vi "FigureExample.vi"() -> ()   [LabVIEW 2021]
doc: "Example of figures classes."
uses:
  Circle/Circle.lvclass
  Rectangle/Rectangle.lvclass
  Square/Square.lvclass
  Figure/Figure.lvclass
panel:
  out "Canva":picture
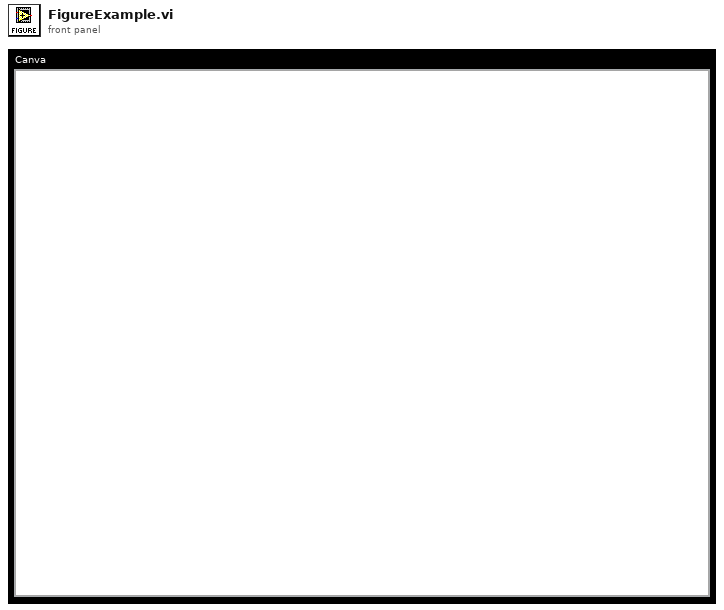
[diagram p1: front panel]
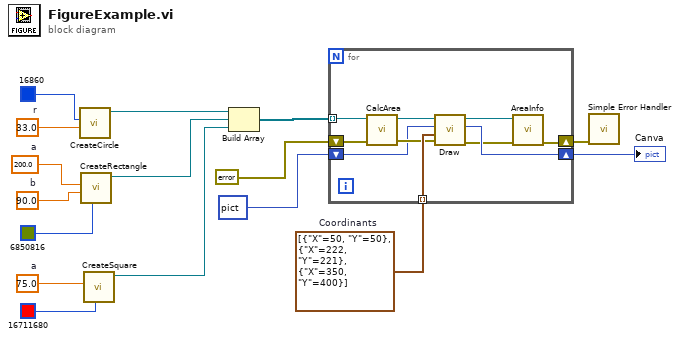
[diagram p0: block diagram]
diagram:
  w3 = cluster{"X":i16, "Y":i16}[] [{"X"=50, "Y"=50}, {"X"=222, "Y"=221}, {"X"=350, "Y"=400}]  # Coordinants
  w10 = 200.0  # a
  w11 = 90.0  # b
  w15 = 33.0  # r
  w16 = 75.0  # a
  n1 = call "CreateCircle.vi"("r"=w15, "Color"=u32 16860) -> ("Circle out"=w9:refnum<class "Circle.lvclass">)  [unwired: 8 in, 1 out]
  n2 = call "CreateRectangle.vi"("Color"=u32 6850816, "b"=w11, "a"=w10) -> ("Rectangle Out"=w8:refnum<class "Rectangle.lvclass">)  [unwired: 7 in, 1 out]
  n3 = call "CreateSquare.vi"("Color"=u32 16711680, "a"=w16) -> ("Square out"=w7:refnum<class "Square.lvclass">)  [unwired: 8 in, 1 out]
  n4 = Build Array(w9, w8, w7) -> (w6:refnum<class "Figure.lvclass">[])
  n5 = for {
    tunnel: w6 -> [w22] mode=indexing
    shift-right: [w26] -> w4
    shift-left: picture data[5B] ("2D Picture In") -> [w19]
    tunnel: w3 -> [w25] mode=indexing
    shift-right: [w18] -> w1
    shift-left: errorcluster {"status"=FALSE, "code"=0, "source"=""} ("Error Out") -> [w17]
    n6 = call-dynamic "CalcArea.vi"("Error In"=w17, "Figure in"=w22) -> ("Error Out"=w20:errorcluster, "Figure out"=w21:refnum<class "Figure.lvclass">)  [unwired: 7 in, 1 out]
    n7 = call-dynamic "Draw.vi"("Error In"=w20, "Coordinants"=w25, "2D Picture In"=w19, "Figure in"=w21) -> ("Error Out"=w24:errorcluster, "2D Picture Out"=w26:picture, "Figure out"=w23:refnum<class "Figure.lvclass">)  [unwired: 5 in]
    n8 = call-dynamic "AreaInfo.vi"("Error In"=w24, "Figure in"=w23) -> ("Error Out"=w18:errorcluster)  [unwired: 8 in, 1 out]
  }
  "Canva" <- w4
  n9 = call <vilib>:"Simple Error Handler.vi"("error in (no error)"=w1) -> ()  [unwired: 4 in, 5 out]
